vi "Convert plane.vi"(7 "File Handle":u32, 8 "error in (no error)":errorcluster, 9 "Frame Index":i32=-1, 10 "file in":path, 11 "Image in":T1) -> (0 "error out":errorcluster, 3 "Image out":T1)   [LabVIEW 2012, in "DAQOrcaFlash.lvclass"]
uses:
  DAQOrcaFlash.lvclass
  <vilib>/vision/Image Controls.llb/IMAQ Image.ctl
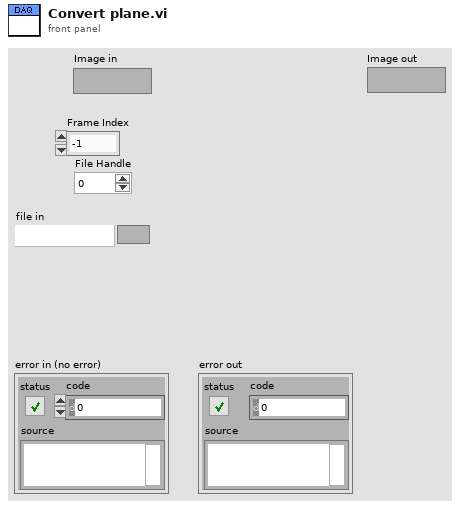
[diagram p1: front panel]
types:
  T1 = typedef "IMAQ Image.ctl" = refnum<image>
  T2 = cluster{"Rows Per Strip":i32, "Photometric":i32, "Compression Type":i32}
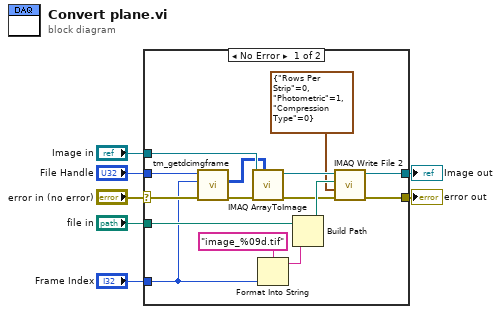
[diagram p0: block diagram]
diagram:
  n1 = case shown="No Error" "error in (no error)" {
    selector: "error in (no error)" -> [w20 w24]
    tunnel: "File Handle" -> [w22 _]
    tunnel: "file in" -> [w14 _]
    tunnel: [w18 w24] -> w5
    tunnel: "Frame Index" -> [w13 _]
    tunnel: "Image in" -> [w19 w23]
    tunnel: [w17 w23] -> w2
    frame No Error {
      n2 = call <userlib>:"tm_getdcimgframe.vi"("error in (no error)"=w20, "Frame Index"=w13, "File Handle in"=w22) -> ("error out"=w10:errorcluster, "Data"=w11:u16[][])  [unwired: 5 in, 2 out]
      n3 = call "IMAQ ArrayToImage"("Image Pixels (U16)"=w11, "error in (no error)"=w10, "Image"=w19) -> ("error out"=w9:errorcluster, "Image Out"=w12:T1)  [unwired: 7 in]
      n4 = Format Into String(format string="image_%09d.tif", w13) -> (resulting string=w15:string)  [unwired: 2 in, 1 out]
      n5 = Build Path(base path=w14, name or relative path=w15) -> (appended path=w21:path)
      n6 = call-poly "IMAQ Write File 2"("error in (no error)"=w9, "TIFF Options"=T2 {"Rows Per Strip"=0, "Photometric"=1, "Compression Type"=0}, "File Path"=w21, "Image"=w12) -> ("error out"=w18:errorcluster, "Image Out (duplicate)"=w17:T1)  [unwired: 6 in]
    }
    frame Error {
    }
  }
  "error out" <- w5
  "Image out" <- w2
